vi "emi_Enum Info.vi"(7 "Enum":variant, 11 "error in (no error)":errorcluster) -> (4 "Text Elements":string[](array[string]), 8 "Numeric Value":u64, 10 "Numb Elements":i32, 15 "error out":errorcluster)   [LabVIEW 2011]
doc: "Return an array of an enums text strings, and the total number of possible values for the enum.\n\nIf another numeric is connected to \"Enum\" Numb Elements will be 0 and the list will be empty. \nIf a non numeric datatype is connected, and error is returned.\n\nHigh Priority\nOn Error: No Actions"
uses:
  <vilib>/Utility/VariantDataType/VariantType.lvlib
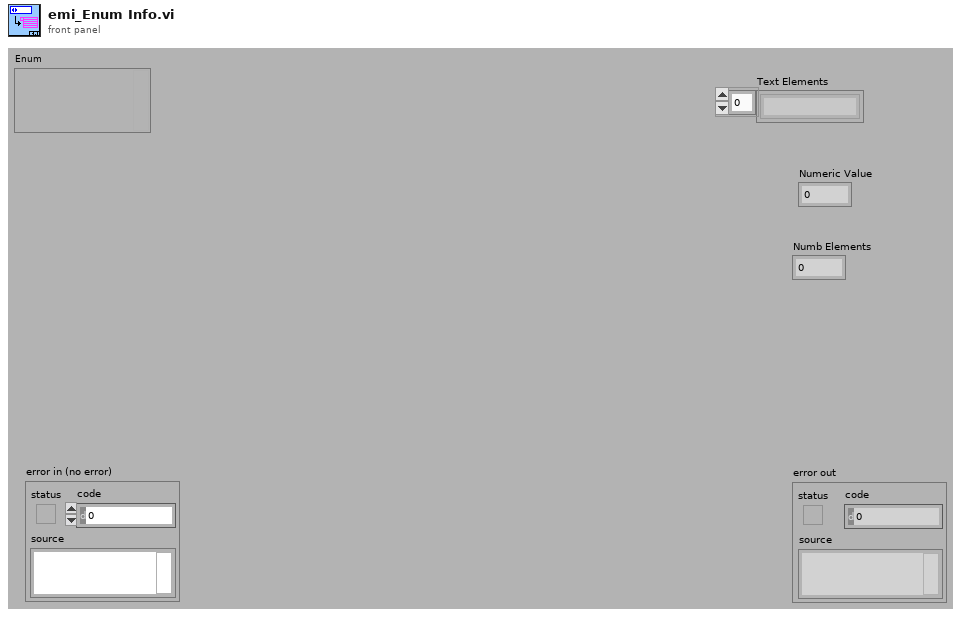
[diagram p1: front panel]
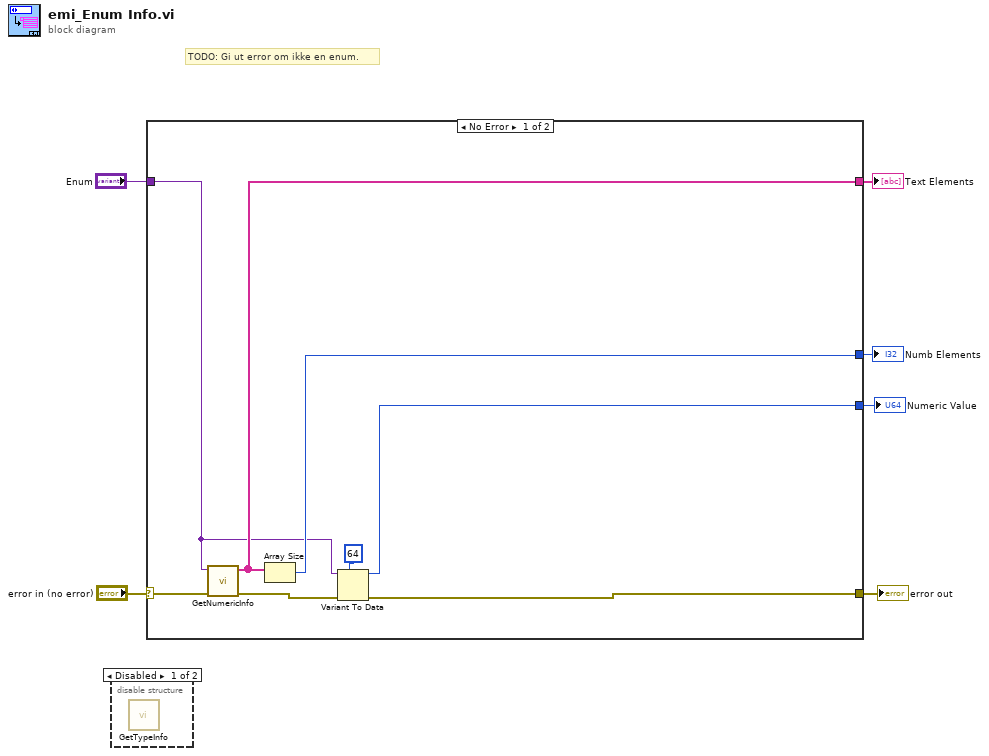
[diagram p0: block diagram]
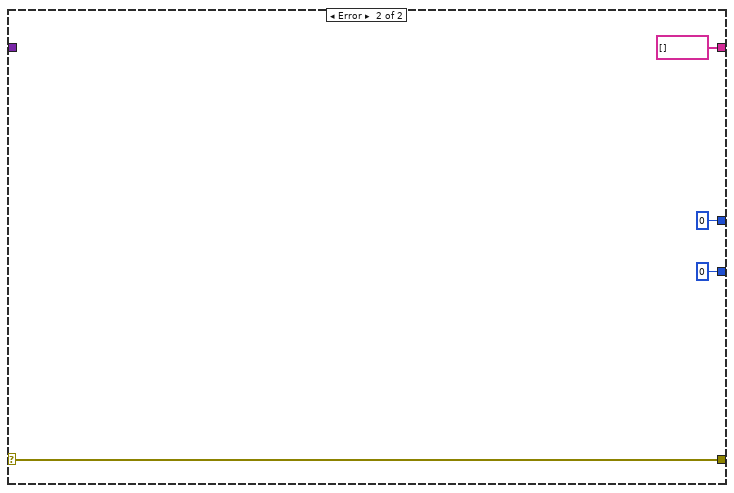
[diagram p3: hidden frame]
diagram:
  # "TODO: Gi ut error om ikke en enum."
  n1 = disable-structure shown="Disabled" {
    frame Disabled {
      n2 = call <vilib>:"GetTypeInfo.vi"() -> ()  [unwired: 7 in, 5 out]
    }
    frame Enabled {
    }
  }
  n3 = case shown="No Error" "error in (no error)" {
    selector: "error in (no error)" -> [w14 w18]
    tunnel: [w9 w18] -> w5
    tunnel: "Enum" -> [w8 _]
    tunnel: [w13 string[] [] ("EnumNames")] -> w2
    tunnel: [w12 0] -> w3
    tunnel: [w7 u64 0] -> w1
    frame No Error {
      n4 = call <vilib>:"GetNumericInfo.vi"("error in (no error)"=w14, "Variant"=w8) -> ("error out"=w10:errorcluster, "EnumNames"=w13:string[])  [unwired: 6 in, 2 out]
      n5 = Array Size(array=w13) -> (size(s)=w12:i32)
      n6 = Variant To Data(error in=w10, type=u64 64, Variant=w8) -> (data=w7:u64, error out=w9:errorcluster)
    }
    frame Error {
    }
  }
  "error out" <- w5
  "Numb Elements" <- w3
  "Text Elements" <- w2
  "Numeric Value" <- w1
